vi "executarTeste.vi"(0 "IP_Servidor":string, 1 "frequencia":dbl format="%#.9f", 2 "executar?":refnum<vi>, 5 "Porta_Servidor":u16, 7 "tamanho":i32=1, 9 "Interações":u32=1000, 11 "error in (no error)":errorcluster) -> (4 "media":dbl, 6 "desvio":dbl, 8 "erro":dbl, 10 "mensagens":i32, 15 "error out":errorcluster)   [LabVIEW 2016]
uses:
  Cliente.lvclass
  <vilib>/Analysis/NI_AALBase.lvlib
panel:
  out "Iteração":i32
  out "msg_enviada":string
  out "msg_recebida":string
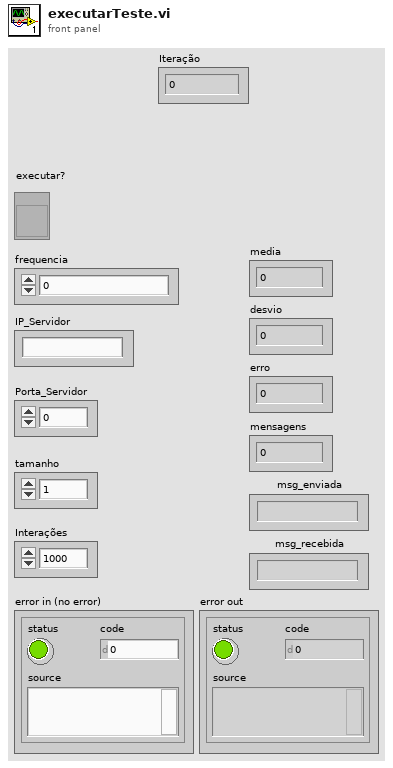
[diagram p1: front panel]
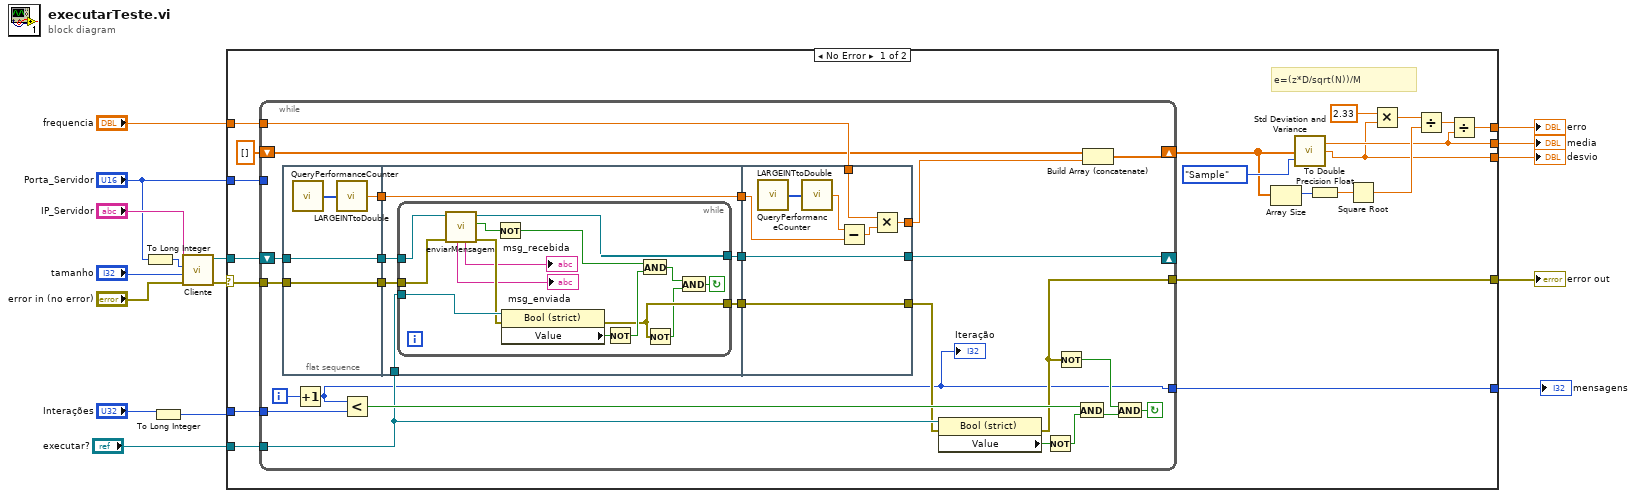
[diagram p0: block diagram]
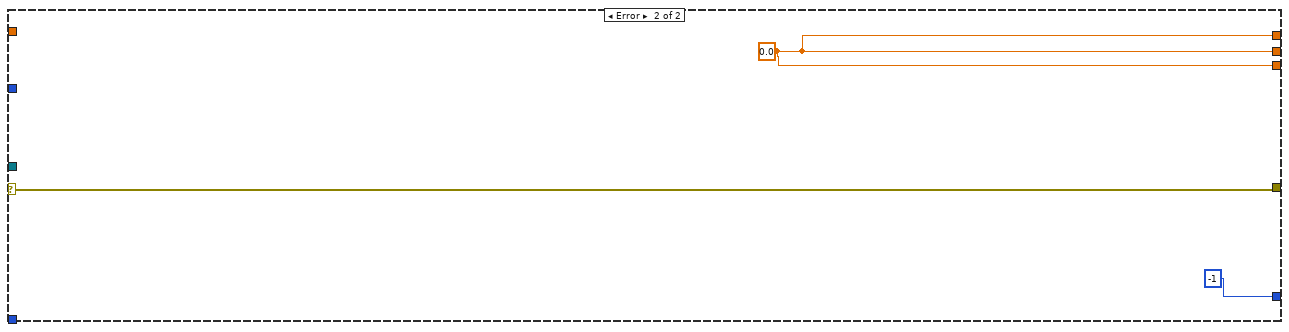
[diagram p2: hidden frame]
diagram:
  n1 = To Long Integer(number="Porta_Servidor") -> (32bit integer=w4:i32)
  n2 = To Long Integer(number="Interações") -> (32bit integer=w1:i32)
  n3 = call "Cliente.vi"("error in (no error)"="error in (no error)", "tmsg"="tamanho", "port"=w4, "addr_srv"="IP_Servidor") -> ("error out"=w10:errorcluster, "Cliente out"=w8:refnum<class "Cliente.lvclass">)  [unwired: 6 in]
  n4 = case shown="No Error" w10 {
    selector: w10 -> [w33 w97]
    tunnel: w1 -> [w36 _]
    tunnel: "Porta_Servidor" -> [w35 _]
    tunnel: w8 -> [w34 _]
    tunnel: "frequencia" -> [w32 _]
    tunnel: [w30 w97] -> w12
    tunnel: [w29 -1] -> w13
    tunnel: [w20 w96] -> w14
    tunnel: [w18 w96] -> w15
    tunnel: [w19 w96] -> w16
    tunnel: "executar?" -> [w24 _]
    frame No Error {
      # "e=(z*D/sqrt(N))/M"
      n5 = while {
        tunnel: w36 -> [w61]
        tunnel: w35 -> [_]
        shift-right: [w39] -> _
        shift-left: w34 -> [w57]
        tunnel: w33 -> [w46]
        tunnel: w32 -> [w51]
        shift-right: [w47] -> w27
        shift-left: dbl[] [] -> [w49]
        tunnel: [w40] -> w30
        tunnel: [w37] -> w29
        tunnel: w24 -> [w45]
        i -> [w38]
        stop <- w43 continue-if-true
        n6 = flat-sequence {
          tunnel: w57 -> [w65]
          tunnel: [w65] -> w56
          tunnel: w46 -> [w64]
          tunnel: [w64] -> w54
          tunnel: [w62] -> w53
          tunnel: w56 -> [w71]
          tunnel: [w70] -> w55
          tunnel: w54 -> [w69]
          tunnel: w53 -> [w68]
          tunnel: [w68] -> w52
          tunnel: [w67] -> w50
          tunnel: w45 -> [w66]
          tunnel: w55 -> [w94]
          tunnel: [w94] -> w39
          tunnel: w52 -> [w91]
          tunnel: w51 -> [w89]
          tunnel: [w88] -> w48
          tunnel: w50 -> [w87]
          tunnel: [w87] -> w44
          frame #0 {
            n7 = call "QueryPerformanceCounter.vi"() -> ("lpPerformanceCount"=w63:u32[])
            n8 = call "LARGEINTtoDouble.vi"("64Bit Number"=w63) -> ("Double Output"=w62:dbl)
          }
          frame #1 {
            n9 = while {
              tunnel: w71 -> [w82]
              tunnel: [w74] -> w70
              tunnel: w69 -> [w81]
              tunnel: [w78] -> w67
              tunnel: w66 -> [w80]
              stop <- w76 continue-if-true
              n10 = call "enviarMensagem.vi"("error in (no error)"=w81, "Cliente in"=w82) -> ("error out"=w79:errorcluster, "ok"=w84:bool, "Cliente out"=w74:refnum<class "Cliente.lvclass">, "msg_recebida"=→"msg_recebida":string, "msg_enviada"=→"msg_enviada":string)  [unwired: 5 in]
              n11 = Not(x=w84) -> (.not. x?=w83:bool)
              n12 = property class="Bool (strict)"(reference=w80, error in=w79) -> (error out=w78:errorcluster, "Value"=w85:bool)  [unwired: 1 out]
              n13 = Not(x=w85) -> (.not. x?=w86:bool)
              n14 = And(x=w83, y=w86) -> (x .and. y?=w75:bool)
              n15 = Not(x=w78) -> (.not. x?=w77:bool)
              n16 = And(x=w75, y=w77) -> (x .and. y?=w76:bool)
            }
          }
          frame #2 {
            n17 = call "QueryPerformanceCounter.vi"() -> ("lpPerformanceCount"=w93:u32[])
            n18 = call "LARGEINTtoDouble.vi"("64Bit Number"=w93) -> ("Double Output"=w92:dbl)
            n19 = Subtract(x=w92, y=w91) -> (x-y=w90:dbl)
            n20 = Multiply(x=w89, y=w90) -> (x*y=w88:dbl)
          }
        }
        n21 = Increment(x=w38) -> (x+1=w37:i32)
        "Iteração" <- w37
        n22 = Less?(x=w37, y=w61) -> (x < y?=w60:bool)
        n23 = property class="Bool (strict)"(reference=w45, error in=w44) -> (error out=w40:errorcluster, "Value"=w59:bool)  [unwired: 1 out]
        n24 = Not(x=w59) -> (.not. x?=w58:bool)
        n25 = Not(x=w40) -> (.not. x?=w41:bool)
        n26 = And(x=w60, y=w58) -> (x .and. y?=w42:bool)
        n27 = Build Array (concatenate)(w49, w48) -> (w47:dbl[])
        n28 = And(x=w41, y=w42) -> (x .and. y?=w43:bool)
      }
      n29 = Array Size(array=w27) -> (size(s)=w23:i32)
      n30 = call <vilib>:"Std Deviation and Variance.vi"("X"=w27, "Weighting (Sample)"=enum16{"Sample", "Population"}."Sample") -> ("mean"=w20:dbl, "standard deviation"=w18:dbl)  [unwired: 1 out]
      n31 = To Double Precision Float(number=w23) -> (double precision float=w22:dbl)
      n32 = Square Root(x=w22) -> (sqrt(x)=w25:dbl)
      n33 = Multiply(x=2.33 ("y"), y=w18) -> (x*y=w26:dbl)
      n34 = Divide(x=w26, y=w25) -> (x/y=w21:dbl)
      n35 = Divide(x=w21, y=w20) -> (x/y=w19:dbl)
    }
    frame Error {
      w96 = 0.0 ("mean")
    }
  }
  "erro" <- w16
  "desvio" <- w15
  "media" <- w14
  "mensagens" <- w13
  "error out" <- w12
